vi "Configure Timebase Basic.vi"(0 "VISA resource name":refnum<visa-resource-name>, 5 "Offset (0)":dbl, 7 "Scale":T1(ring)=enum."50us", 9 "Mode (0: Main)":i32(ring) items=["Main", "XY", "Roll"], 11 "error in (no error)":errorcluster) -> (4 "VISA resource name out":refnum<visa-resource-name>, 15 "error out":errorcluster)   [LabVIEW 2015]
doc: "Configures the basic setting for timebase."
uses:
  ZhiYuan ZDS Series for TCP.lvlib
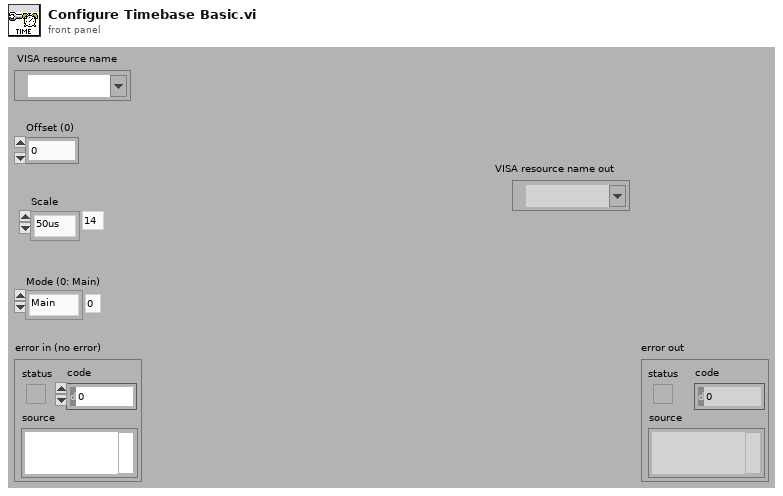
[diagram p1: front panel]
types:
  T1 = enum16{"1ns", "2ns", "5ns", "10ns", "20ns", "50ns", "100ns", "200ns", "500ns", "1us", "2us", "5us", "10us", "20us", "50us", "100us", "200us", "500us", "1ms", "2ms", "5ms", "10ms", "20ms", "50ms", "100ms", "200ms", "500ms", "1s", "2s", "5s", "10s", "20s", "50s", "100s"}
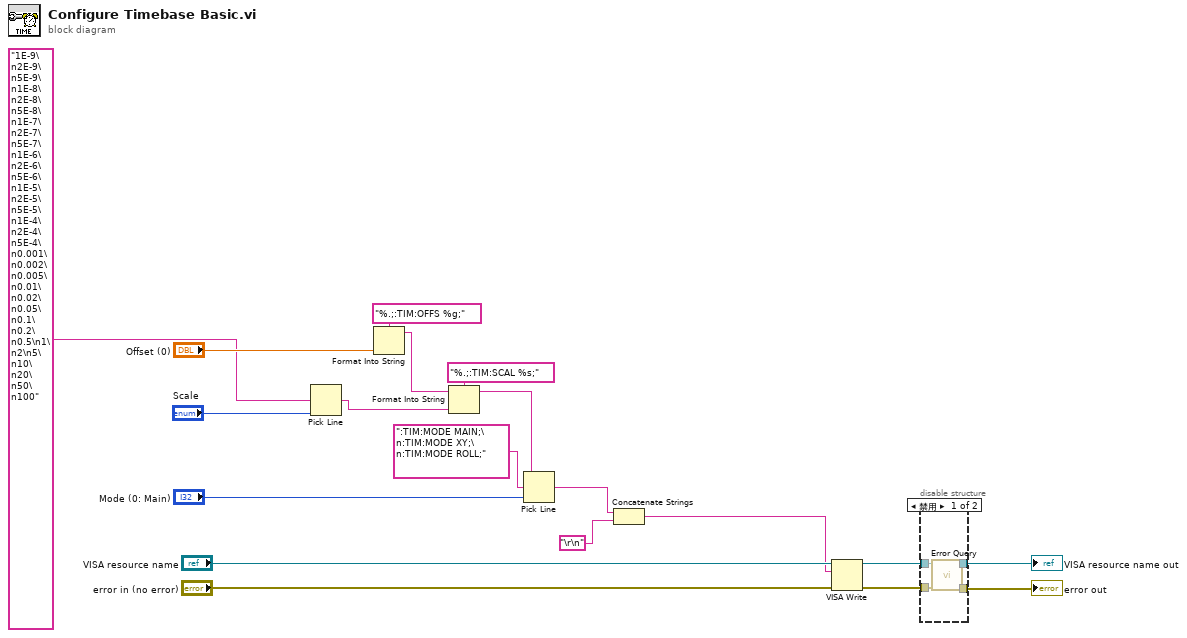
[diagram p0: block diagram]
diagram:
  n1 = Pick Line(multi-line string="1E-9\n2E-9\n5E-9\n1E-8\n2E-8\n5E-8\n1E-7\n2E-7\n5E-7\n1E-6\n2E-6\n5E-6\n1E-5\n2E-5\n5E-5\n1E-4\n2E-4\n5E-4\n0.001\n0.002\n0.005\n0.01\n0.02\n0.05\n0.1\n0.2\n0.5\n1\n2\n5\n10\n20\n50\n100", line index="Scale") -> (output string=w5:string)  [unwired: 1 in]
  n2 = Format Into String(format string="%.;:TIM:OFFS %g;", "Offset (0)") -> (resulting string=w17:string)  [unwired: 2 in, 1 out]
  n3 = Format Into String(format string="%.;:TIM:SCAL %s;", initial string=w17, w5) -> (resulting string=w13:string)  [unwired: 1 in, 1 out]
  n4 = Pick Line(string ("")=w13, multi-line string=":TIM:MODE MAIN;\n:TIM:MODE XY;\n:TIM:MODE ROLL;", line index="Mode (0: Main)") -> (output string=w4:string)
  n5 = Concatenate Strings(w4, "\r\n") -> (w2:string)
  n6 = VISA Write(VISA resource name="VISA resource name", write buffer=w2, error in (no error)="error in (no error)") -> (VISA resource name out=w10:refnum<visa-resource-name>, error out=w9:errorcluster)  [unwired: 1 out]
  n7 = disable-structure shown="禁用" {
    disable-tunnel: w10 -> [w23 w24]
    disable-tunnel: w9 -> [w22 w25]
    disable-tunnel: [w21 w24] -> w8
    disable-tunnel: [w20 w25] -> w7
    frame Disabled {
      n8 = call "Error Query.vi"("error in (no error)"=w22, "VISA resource name"=w23) -> ("error out"=w20:errorcluster, "VISA resource name out"=w21:refnum<visa-resource-name>)  [unwired: 6 in, 2 out]
    }
    frame Enabled {
    }
  }
  "VISA resource name out" <- w8
  "error out" <- w7
